vi "ILABs_RemoteCommandHandler.vi"(2 "error In":errorcluster, 4 "data":string, 5 "action":string) -> (0 "errorOut":string, 1 "response":string)   [LabVIEW 2009]
panel:
  out "Control":bool
  out "Connection Status":string
  in  "Case Constant\n(See Context Help)":bool=TRUE
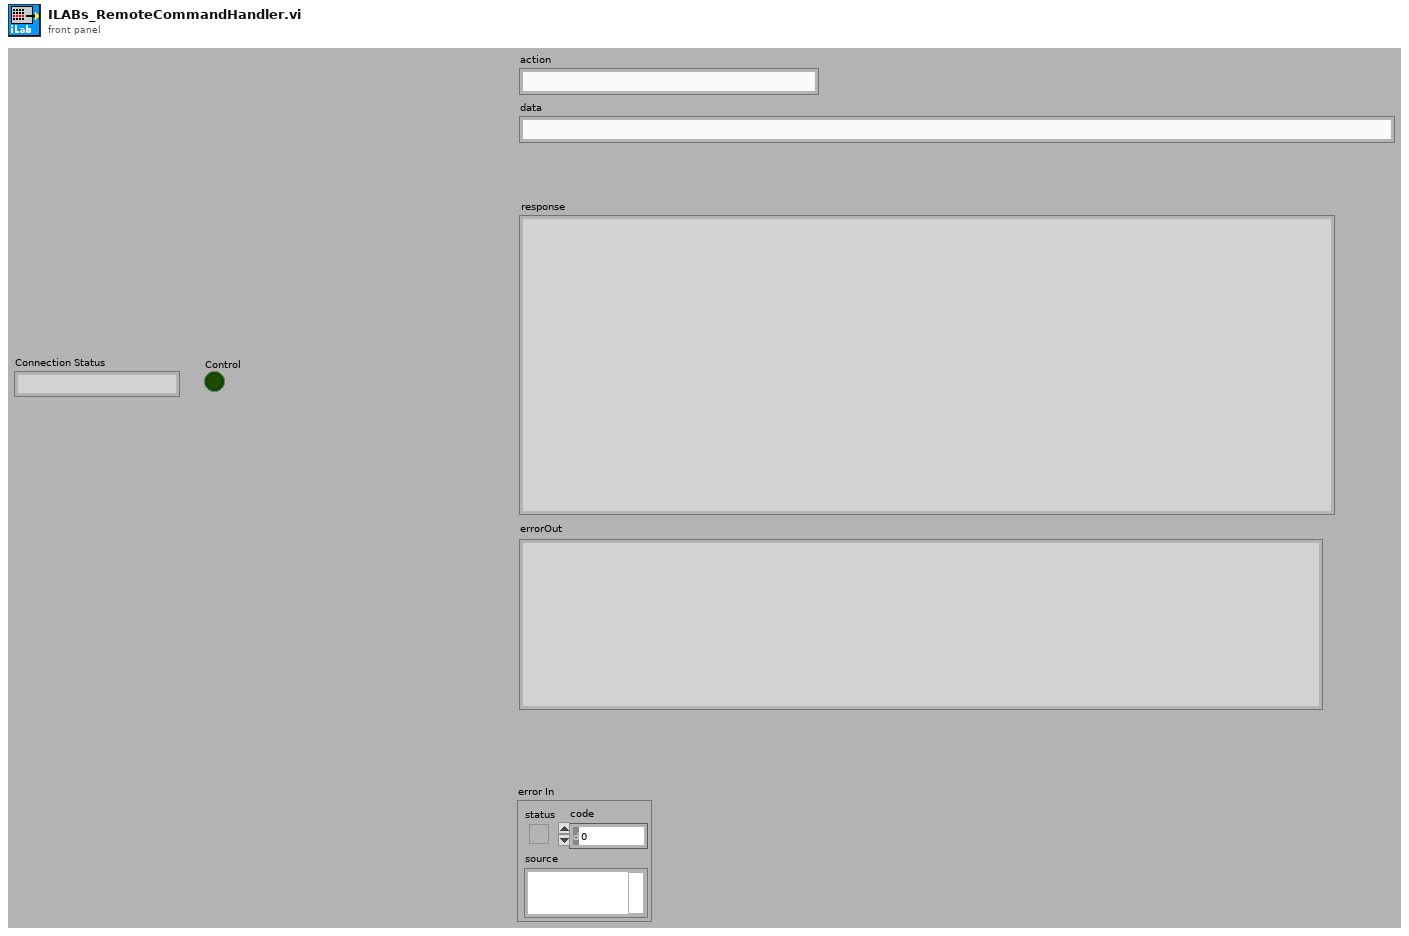
[diagram p1: front panel]
types:
  T1 = typedef "LVRemotePanelConnectionsTypeDef.ctl" = cluster{"VI Name":string, "Remote":string, "UserName":string, "Port":i32, "Status":enum32{"Viewing", "Waiting For Control", "Controlling"}, "Create Time":timestamp, "Status Time":timestamp, "Control End Time":timestamp}[]
  T2 = cluster{"VI Name":string, "Remote":string, "UserName":string, "Port":i32, "Status":enum32{"Viewing", "Waiting For Control", "Controlling"}, "Create Time":timestamp, "Status Time":timestamp, "Control End Time":timestamp}
  T3 = enum32{"Viewing", "Waiting For Control", "Controlling"}
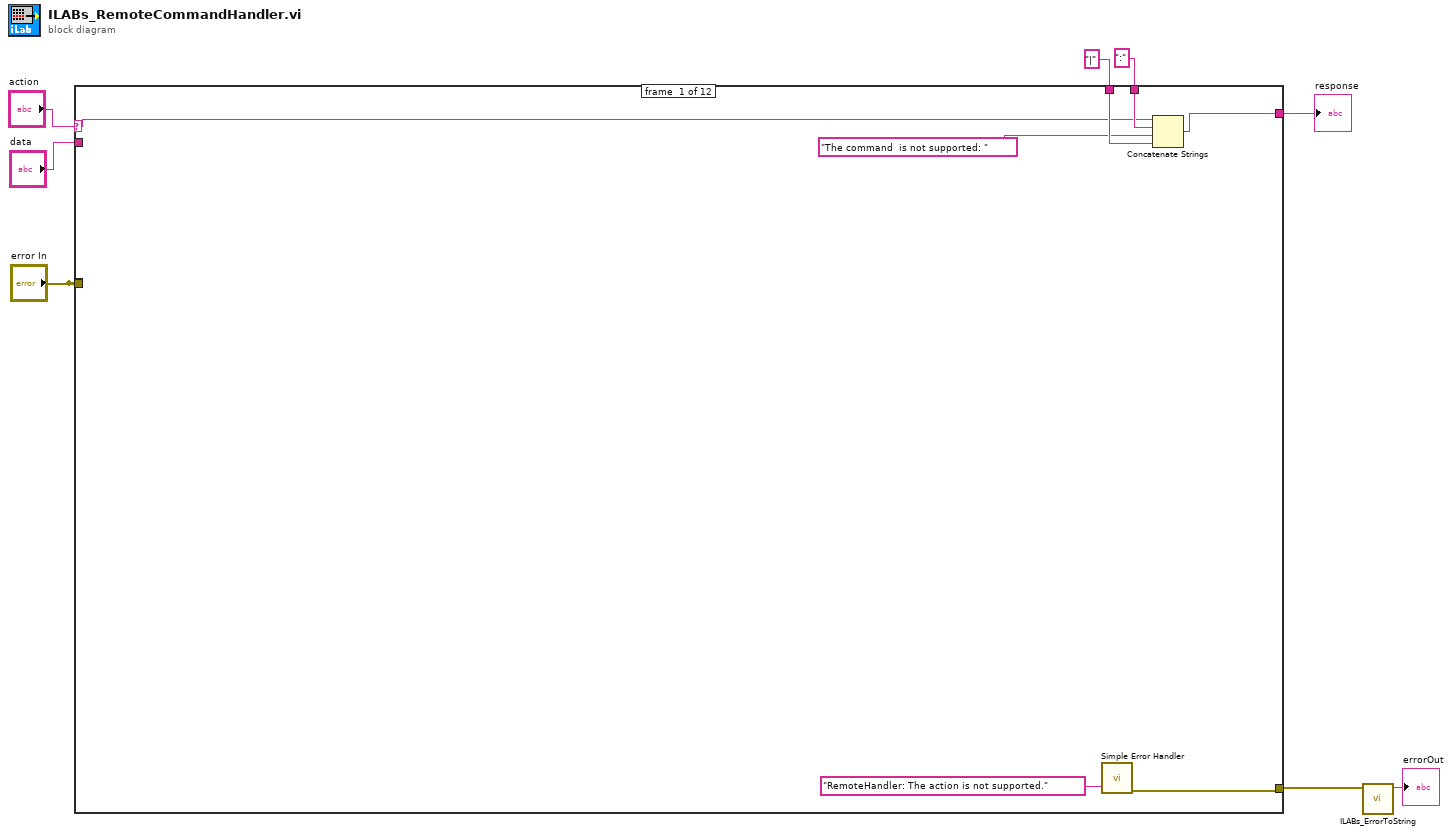
[diagram p0: block diagram]
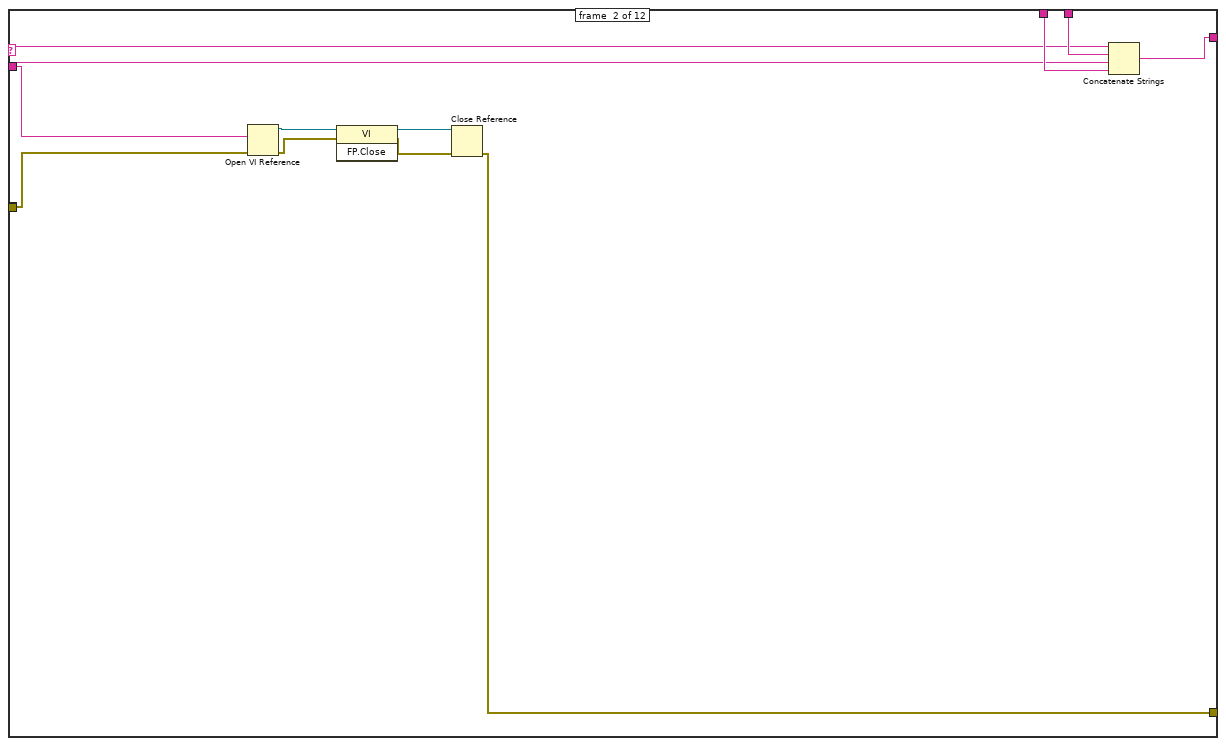
[diagram p2: hidden frame]
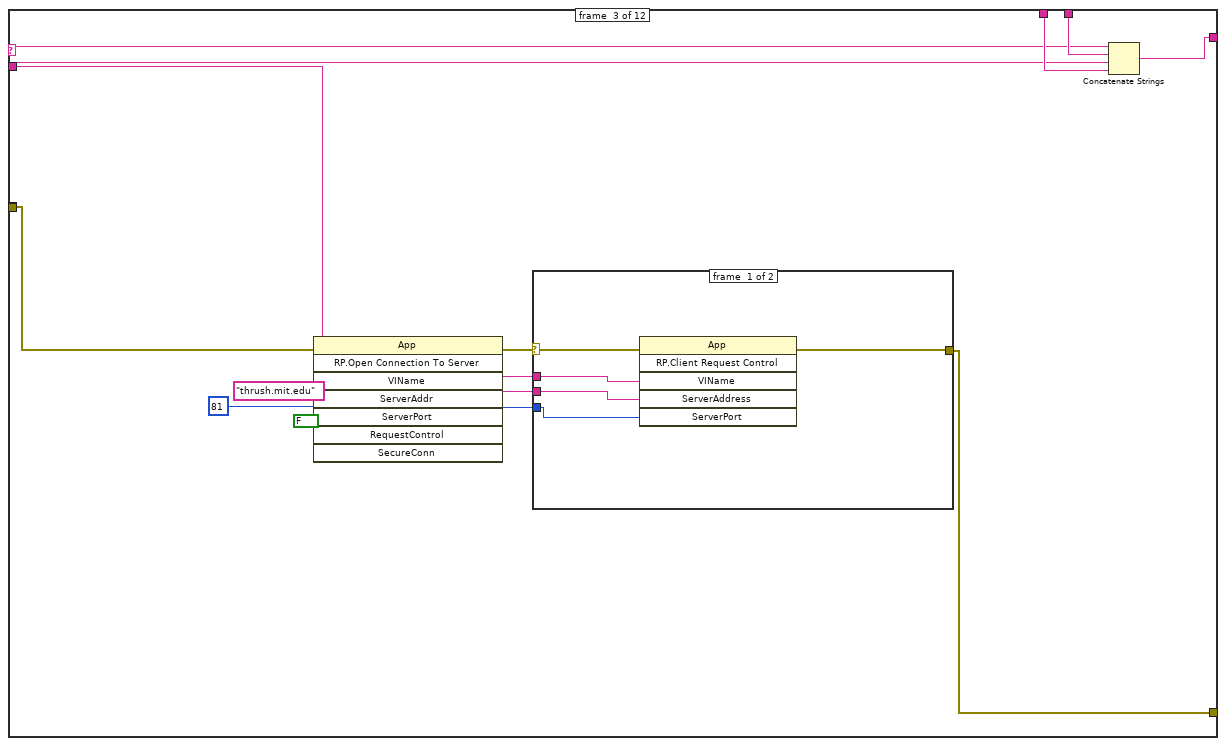
[diagram p3: hidden frame]
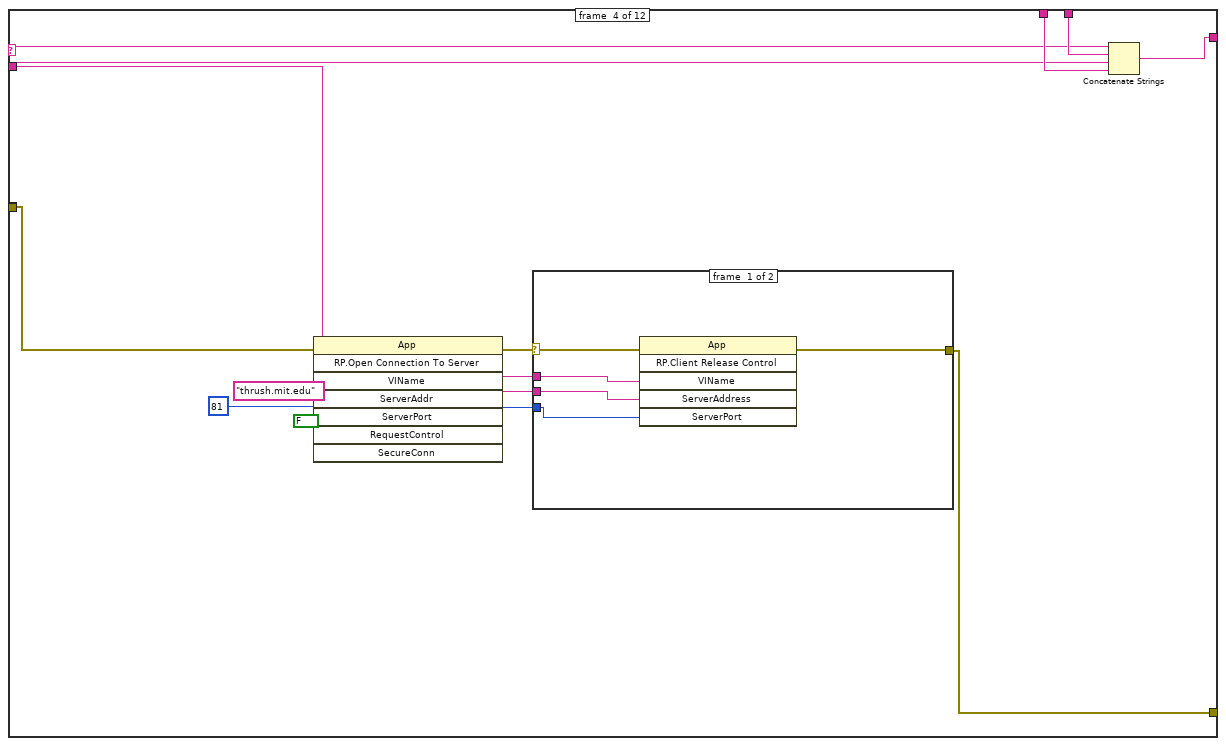
[diagram p5: hidden frame]
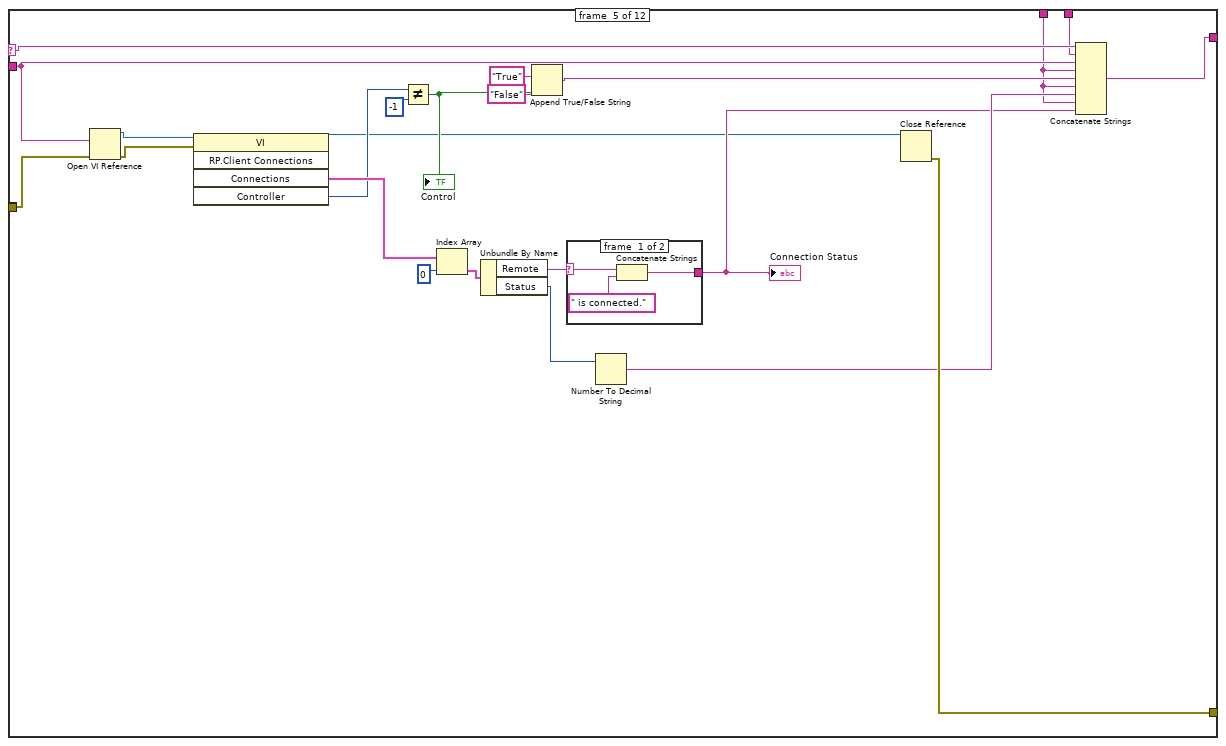
[diagram p7: hidden frame]
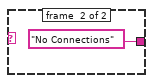
[diagram p8: hidden frame]
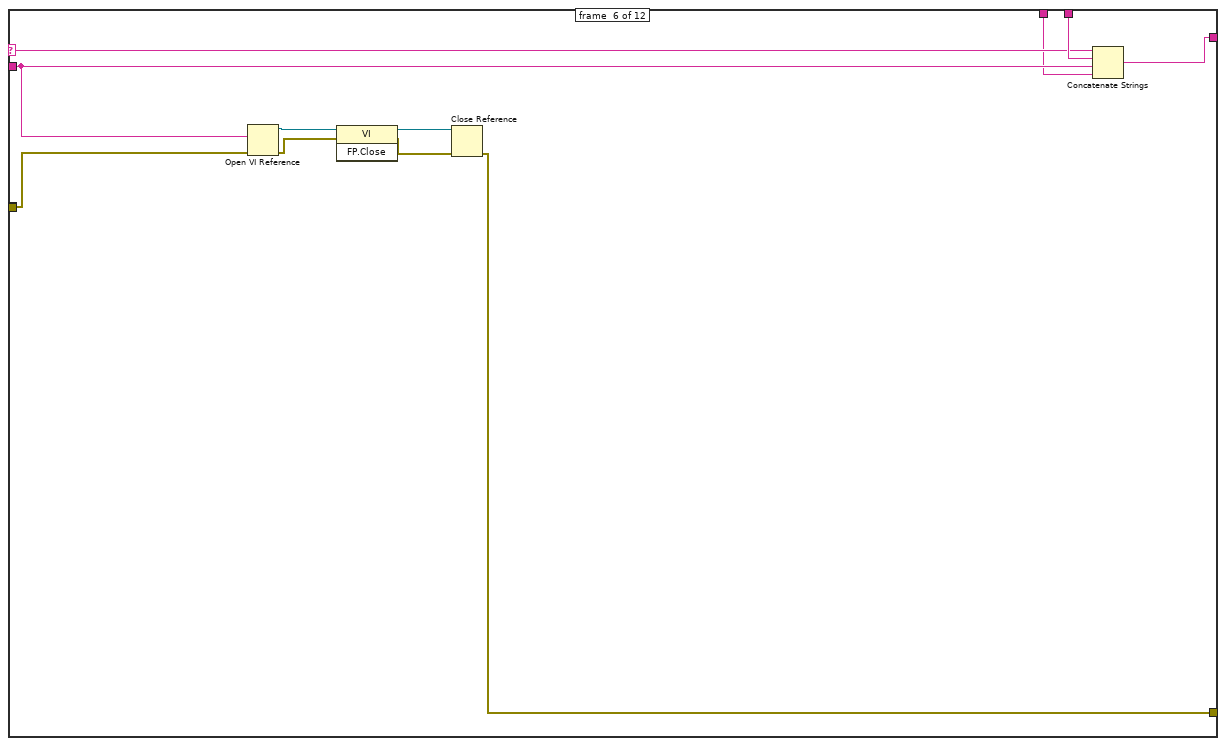
[diagram p9: hidden frame]
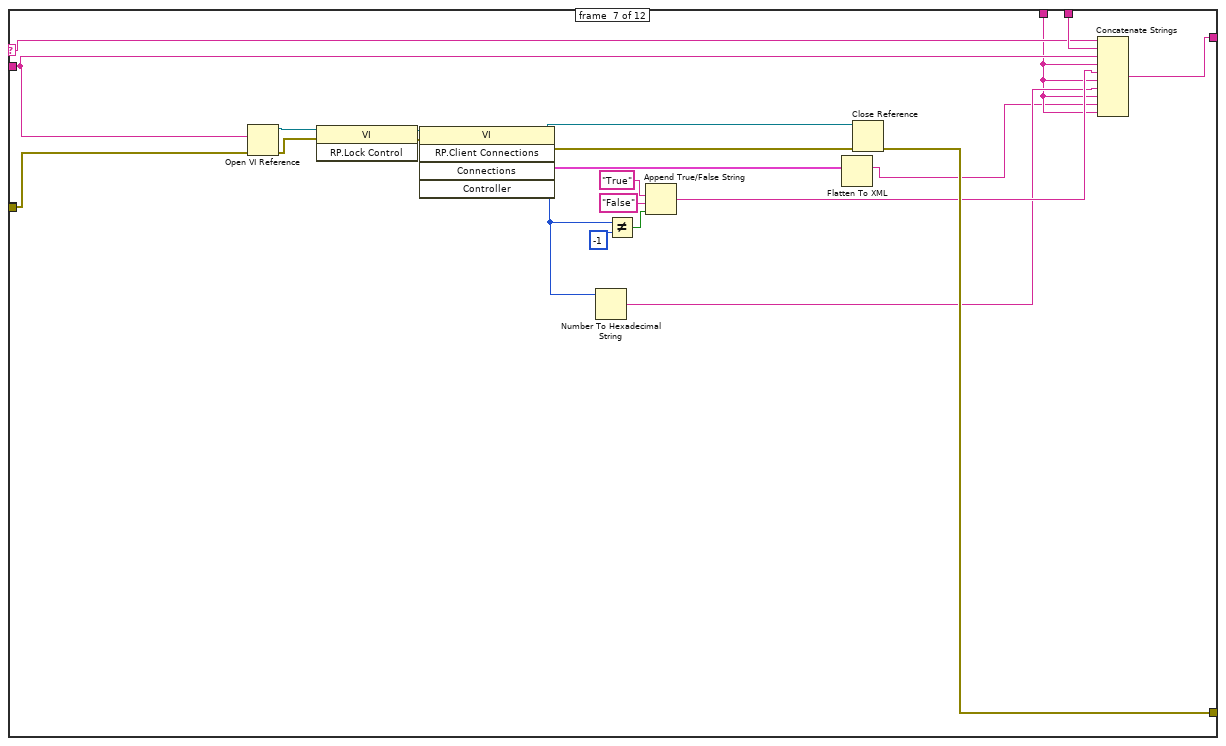
[diagram p10: hidden frame]
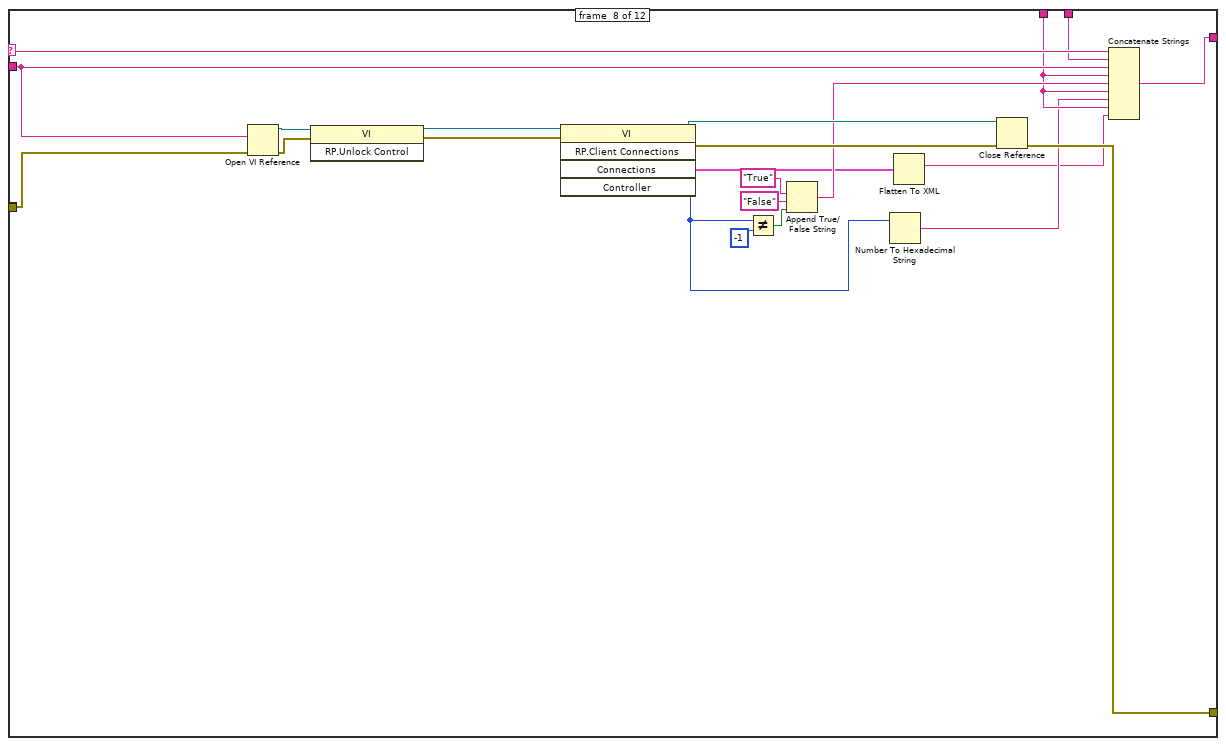
[diagram p11: hidden frame]
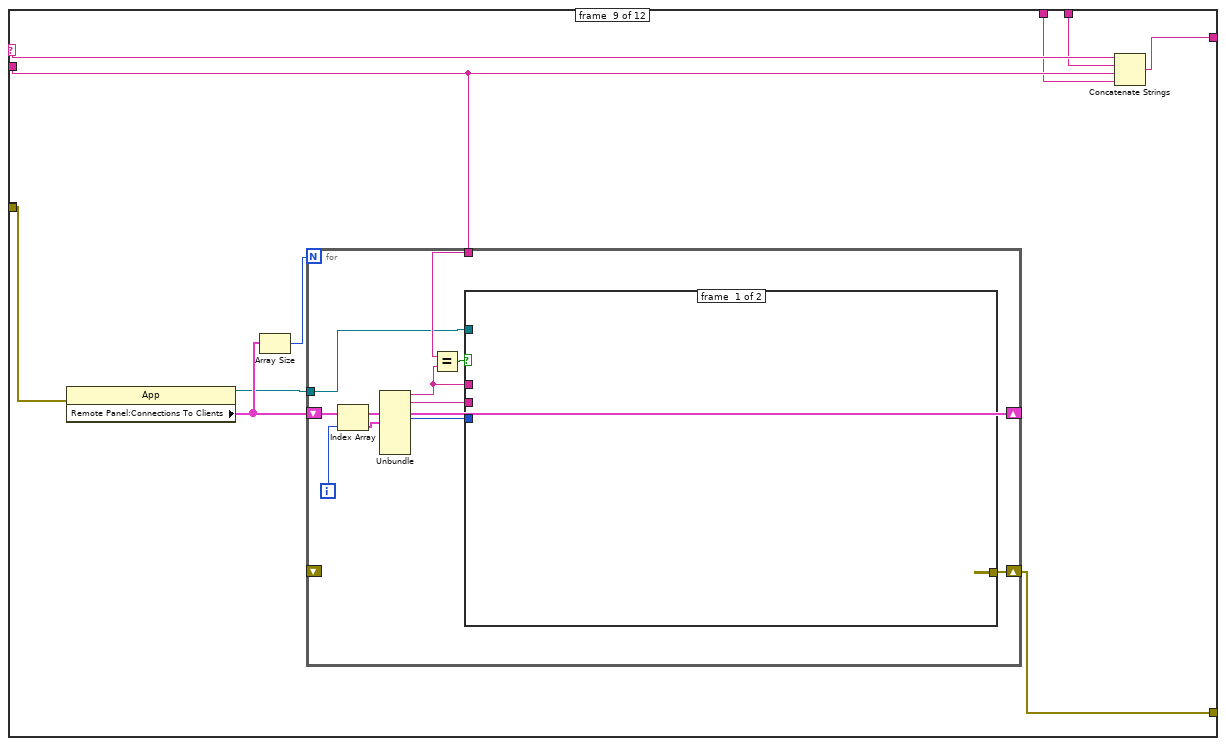
[diagram p12: hidden frame]
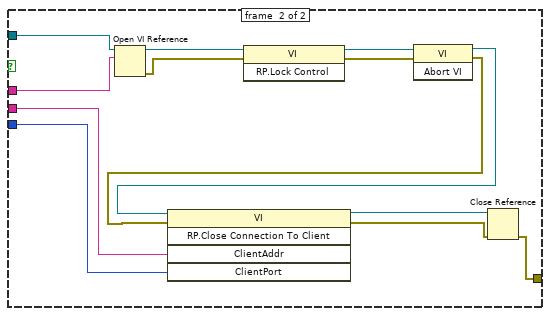
[diagram p13: hidden frame]
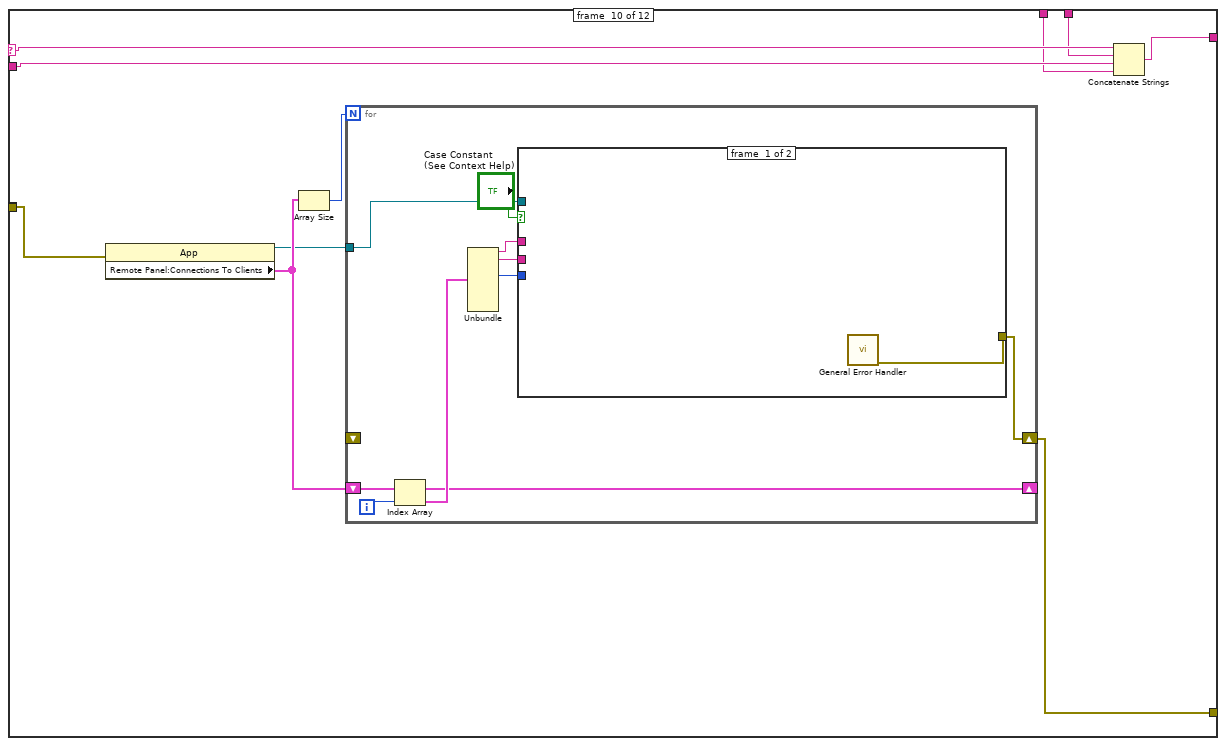
[diagram p14: hidden frame]
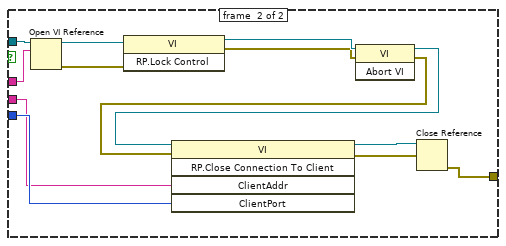
[diagram p15: hidden frame]
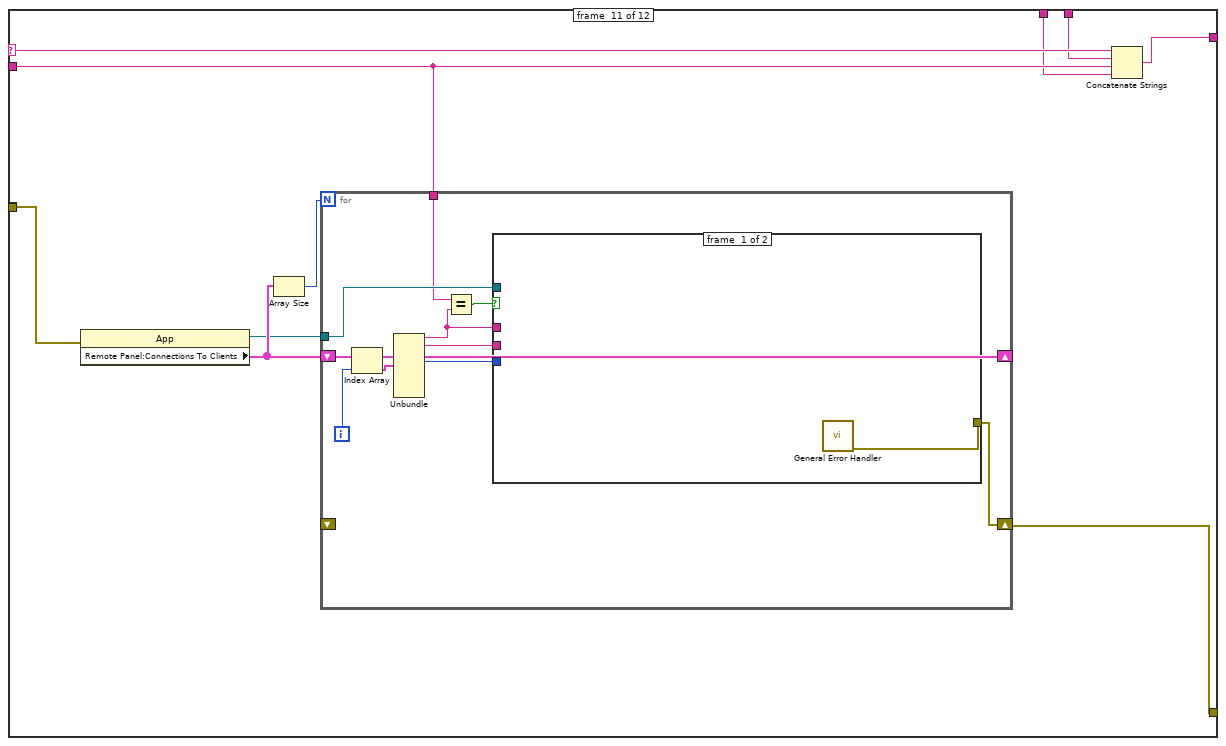
[diagram p16: hidden frame]
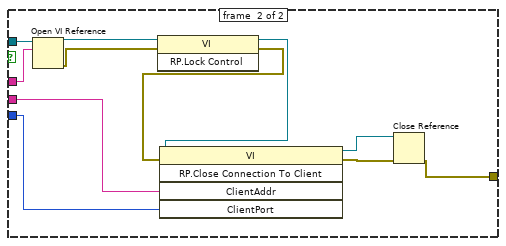
[diagram p17: hidden frame]
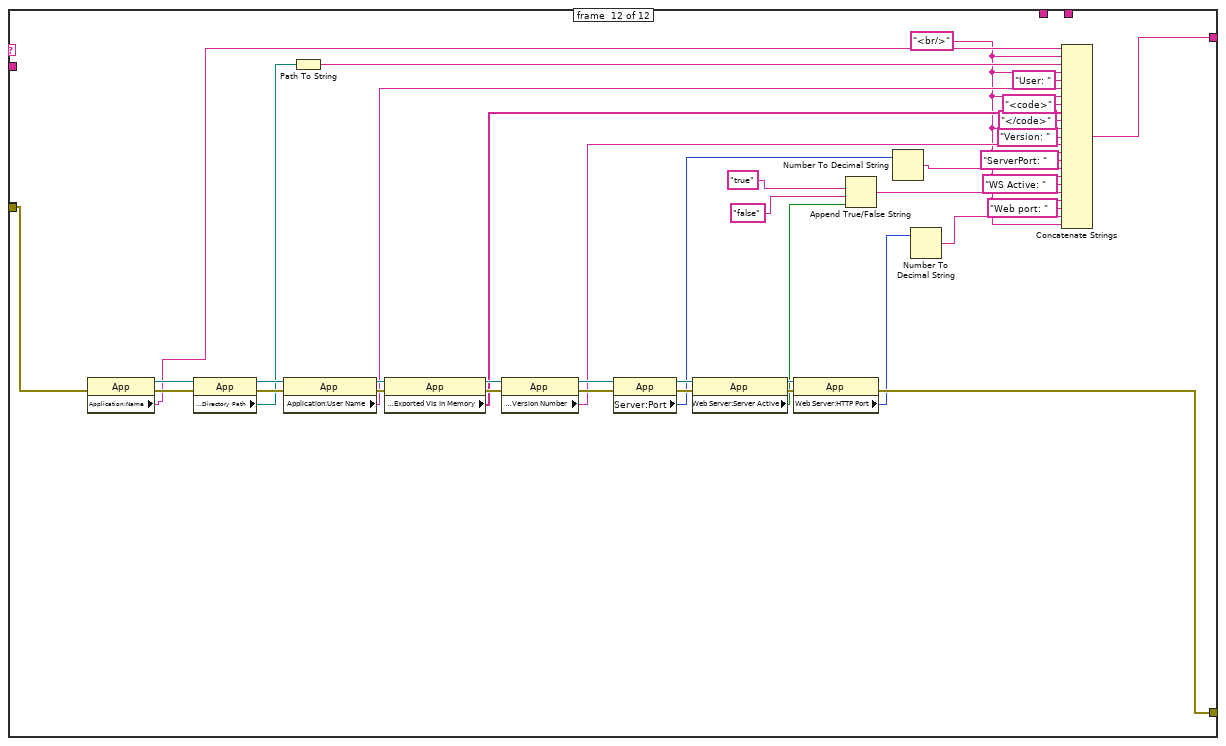
[diagram p18: hidden frame]
diagram:
  n1 = case shown="\"appStatus\"" "action" {
    selector: "action" -> [w9 w17 w34 w51 w67 w90 w107 w129 w146 w179 w212 _]
    tunnel: "data" -> [_ w16 w29 w46 w66 w89 w106 w128 w145 w178 w211 _]
    tunnel: [w15 w20 w37 w54 w81 w92 w116 w138 w152 w183 w218 w241] -> w7
    tunnel: [w13 w21 w28 w45 w82 w93 w117 w139 w147 w182 w213 w264] -> w5
    tunnel: "error In" -> [_ w22 w27 w44 w83 w94 w118 w140 w148 w181 w214 w279]
    tunnel: "error In" -> [_ _ _ _ _ _ _ _ _ _ _ _]
    tunnel: ":" -> [w12 w18 w35 w52 w62 w91 w108 w127 w144 w177 w210 _]
    tunnel: "|" -> [w11 w19 w36 w53 w61 w88 w102 w125 w143 w176 w209 _]
    frame #0 {
      (unwired) "The" ("message")
      n2 = call <vilib>:"Simple Error Handler.vi"("error source (\" \")"="RemoteHandler: The action is not supported." ("error source (\" \")")) -> ("error out"=w13:errorcluster)  [unwired: 2 in, 6 out]
      n3 = Concatenate Strings(w9, w12, "The command  is not supported: " ("string"), w11) -> (w15:string)
    }
    frame #1 {
      n4 = Open VI Reference(vi path=w16, error in (no error)=w22) -> (vi reference=w26:refnum<vi>, error out=w25:errorcluster)  [unwired: 4 out]
      n5 = invoke class="VI" method="FP.Close"(reference=w26, error in=w25) -> (reference out=w24:refnum<vi>, error out=w23:errorcluster)  [unwired: 1 in, 1 out]
      n6 = Close Reference(reference=w24, error in (no error)=w23) -> (error out=w21:errorcluster)
      n7 = Concatenate Strings(w17, w18, w16, w19) -> (w20:string)
    }
    frame #2 {
      w31 = 81 ("Server Port")
      w32 = "thrush.mit.edu" ("Server Address")
      n8 = invoke class="App" method="RP.Open Connection To Server"(error in=w27, "VIName"=w29, "ServerAddr"=w32, "ServerPort"=w31, "RequestControl"=FALSE ("Request Control")) -> (error out=w30:errorcluster)  [unwired: 3 in, 7 out]
      n9 = case shown="No Error" w30 {
        selector: w30 -> [w42 w43]
        tunnel: w29 -> [w41 _]
        tunnel: w32 -> [w40 _]
        tunnel: w31 -> [w39 _]
        tunnel: [w38 w43] -> w28
        frame #0 {
          n10 = invoke class="App" method="RP.Client Request Control"(error in=w42, "VIName"=w41, "ServerAddress"=w40, "ServerPort"=w39) -> (error out=w38:errorcluster)  [unwired: 2 in, 5 out]
        }
        frame #1 {
        }
      }
      n11 = Concatenate Strings(w34, w35, w29, w36) -> (w37:string)
    }
    frame #3 {
      w48 = 81 ("Server Port")
      w49 = "thrush.mit.edu" ("Server Address")
      n12 = invoke class="App" method="RP.Open Connection To Server"(error in=w44, "VIName"=w46, "ServerAddr"=w49, "ServerPort"=w48, "RequestControl"=FALSE ("Request Control")) -> (error out=w47:errorcluster)  [unwired: 3 in, 7 out]
      n13 = case shown="No Error" w47 {
        selector: w47 -> [w59 w60]
        tunnel: w46 -> [w58 _]
        tunnel: w49 -> [w57 _]
        tunnel: w48 -> [w56 _]
        tunnel: [w55 w60] -> w45
        frame #0 {
          n14 = invoke class="App" method="RP.Client Release Control"(error in=w59, "VIName"=w58, "ServerAddress"=w57, "ServerPort"=w56) -> (error out=w55:errorcluster)  [unwired: 2 in, 5 out]
        }
        frame #1 {
        }
      }
      n15 = Concatenate Strings(w51, w52, w46, w53) -> (w54:string)
    }
    frame #4 {
      n16 = Open VI Reference(vi path=w66, error in (no error)=w83) -> (vi reference=w73:refnum<vi>, error out=w74:errorcluster)  [unwired: 4 out]
      n17 = invoke class="VI" method="RP.Client Connections"(reference=w73, error in=w74) -> (reference out=w63:refnum<vi>, "Connections"=w80:T1, "Controller"=w77:i32)  [unwired: 3 in, 2 out]
      n18 = Not Equal?(x=w77, y=-1) -> (x != y?=w72:bool)
      "Control" <- w72
      n19 = Index Array(array=w80, index=0) -> (element=w75:T2)
      n20 = Unbundle By Name(w75) -> ("Remote"=w78:string, "Status"=w68:T3)
      n21 = Append True/False String(1:w72, 2:"False" ("false string"), 3:"True" ("true string")) -> (0:w69:string)  [unwired: 1 out]
      n22 = case shown="\"\"" w78 {
        selector: w78 -> [w86 _]
        tunnel: [w84 "No Connections"] -> w64
        frame #0 {
          n23 = Concatenate Strings(w86, " is connected." ("string")) -> (w84:string)
        }
        frame #1 {
        }
      }
      "Connection Status" <- w64
      n24 = Number To Decimal String(number=w68) -> (decimal integer string=w65:string)  [unwired: 1 out]
      n25 = Close Reference(reference=w63) -> (error out=w82:errorcluster)  [unwired: 1 in]
      n26 = Concatenate Strings(w67, w62, w66, w61, w69, w61, w65, w61, w64) -> (w81:string)
    }
    frame #5 {
      n27 = Open VI Reference(vi path=w89, error in (no error)=w94) -> (vi reference=w98:refnum<vi>, error out=w97:errorcluster)  [unwired: 4 out]
      n28 = invoke class="VI" method="FP.Close"(reference=w98, error in=w97) -> (reference out=w96:refnum<vi>, error out=w95:errorcluster)  [unwired: 1 in, 1 out]
      n29 = Close Reference(reference=w96, error in (no error)=w95) -> (error out=w93:errorcluster)
      n30 = Concatenate Strings(w90, w91, w89, w88) -> (w92:string)
    }
    frame #6 {
      n31 = Open VI Reference(vi path=w106, error in (no error)=w118) -> (vi reference=w120:refnum<vi>, error out=w119:errorcluster)  [unwired: 4 out]
      n32 = invoke class="VI" method="RP.Lock Control"(reference=w120, error in=w119) -> (reference out=w114:refnum<vi>, error out=w113:errorcluster)  [unwired: 1 in, 1 out]
      n33 = invoke class="VI" method="RP.Client Connections"(reference=w114, error in=w113) -> (reference out=w101:refnum<vi>, error out=w115:errorcluster, "Connections"=w99:T1, "Controller"=w104:i32)  [unwired: 3 in, 1 out]
      n34 = Number To Hexadecimal String(2:w104) -> (0:w103:string)  [unwired: 1 out]
      n35 = Not Equal?(x=w104, y=-1) -> (x != y?=w111:bool)
      n36 = Append True/False String(1:w111, 2:"False" ("false string"), 3:"True" ("true string")) -> (0:w105:string)  [unwired: 1 out]
      n37 = Flatten To XML(anything=w99) -> (xml string=w100:string)
      n38 = Close Reference(reference=w101, error in (no error)=w115) -> (error out=w117:errorcluster)
      n39 = Concatenate Strings(w107, w108, w106, w102, w105, w102, w103, w102, w100, w102) -> (w116:string)
    }
    frame #7 {
      n40 = Open VI Reference(vi path=w128, error in (no error)=w140) -> (vi reference=w142:refnum<vi>, error out=w141:errorcluster)  [unwired: 4 out]
      n41 = invoke class="VI" method="RP.Unlock Control"(reference=w142, error in=w141) -> (reference out=w131:refnum<vi>, error out=w130:errorcluster)  [unwired: 1 in, 1 out]
      n42 = invoke class="VI" method="RP.Client Connections"(reference=w131, error in=w130) -> (reference out=w132:refnum<vi>, error out=w133:errorcluster, "Connections"=w122:T1, "Controller"=w124:i32)  [unwired: 3 in, 1 out]
      n43 = Not Equal?(x=w124, y=-1) -> (x != y?=w136:bool)
      n44 = Append True/False String(1:w136, 2:"False" ("false string"), 3:"True" ("true string")) -> (0:w126:string)  [unwired: 1 out]
      n45 = Number To Hexadecimal String(2:w124) -> (0:w123:string)  [unwired: 1 out]
      n46 = Flatten To XML(anything=w122) -> (xml string=w121:string)
      n47 = Close Reference(reference=w132, error in (no error)=w133) -> (error out=w139:errorcluster)
      n48 = Concatenate Strings(w129, w127, w128, w125, w126, w125, w123, w125, w121) -> (w138:string)
    }
    frame #8 {
      n49 = property class="App"(error in=w148) -> (reference out=w149:refnum<vi>, "Remote Panel:Connections To Clients"=w150:T1)  [unwired: 1 in, 1 out]
      n50 = Array Size(array=w150) -> (size(s)=w151:i32)
      n51 = for {
        N: w151 -> [_]
        shift-right: [w154] -> _
        shift-left: w150 -> [w154]
        tunnel: w145 -> [w160]
        shift-right: [w156] -> w147
        shift-left: _ -> [_]
        tunnel: w149 -> [w153]
        i -> [w162]
        n52 = Index Array(array=w154, index=w162) -> (element=w161:T2)
        n53 = Unbundle(w161) -> ("VI Name"=w155:string, "Remote"=w157:string, "Port"=w158:i32)  [unwired: 5 out]
        n54 = Equal?(x=w160, y=w155) -> (x = y?=w159:bool)
        n55 = case shown="True" w159 {
          tunnel: w158 -> [_ w175]
          tunnel: w157 -> [_ w174]
          tunnel: [_ w173] -> w156
          tunnel: w155 -> [_ w172]
          tunnel: w153 -> [_ w163]
          frame #0 {
          }
          frame #1 {
            n56 = Open VI Reference(application reference (local)=w163, vi path=w172) -> (vi reference=w171:refnum<vi>, error out=w170:errorcluster)  [unwired: 1 in, 3 out]
            n57 = invoke class="VI" method="RP.Lock Control"(reference=w171, error in=w170) -> (reference out=w169:refnum<vi>, error out=w168:errorcluster)  [unwired: 1 in, 1 out]
            n58 = invoke class="VI" method="Abort VI"(reference=w169, error in=w168) -> (reference out=w165:refnum<vi>, error out=w167:errorcluster)  [unwired: 1 in, 1 out]
            n59 = invoke class="VI" method="RP.Close Connection To Client"(reference=w165, error in=w167, "ClientAddr"=w174, "ClientPort"=w175) -> (reference out=w164:refnum<vi>, error out=w166:errorcluster)  [unwired: 1 in, 3 out]
            n60 = Close Reference(reference=w164, error in (no error)=w166) -> (error out=w173:errorcluster)
          }
        }
      }
      n61 = Concatenate Strings(w146, w144, w145, w143) -> (w152:string)
    }
    frame #9 {
      n62 = property class="App"(error in=w181) -> (reference out=w180:refnum<vi>, "Remote Panel:Connections To Clients"=w184:T1)  [unwired: 1 in, 1 out]
      n63 = Array Size(array=w184) -> (size(s)=w185:i32)
      n64 = for {
        N: w185 -> [_]
        shift-right: [w188] -> _
        shift-left: w184 -> [w188]
        shift-right: [w190] -> w182
        shift-left: _ -> [_]
        tunnel: w180 -> [w186]
        i -> [w194]
        n65 = Index Array(array=w188, index=w194) -> (element=w193:T2)
        n66 = Unbundle(w193) -> ("VI Name"=w189:string, "Remote"=w191:string, "Port"=w192:i32)  [unwired: 5 out]
        n67 = case shown="True" "Case Constant\n(See Context Help)" {
          tunnel: w192 -> [_ w208]
          tunnel: w191 -> [_ w207]
          tunnel: [w195 w206] -> w190
          tunnel: w189 -> [_ w205]
          tunnel: w186 -> [_ w196]
          frame #0 {
            n68 = call <vilib>:"General Error Handler.vi"() -> ("error out"=w195:errorcluster)  [unwired: 2 in, 13 out]
          }
          frame #1 {
            n69 = Open VI Reference(application reference (local)=w196, vi path=w205) -> (vi reference=w200:refnum<vi>, error out=w199:errorcluster)  [unwired: 1 in, 3 out]
            n70 = invoke class="VI" method="RP.Lock Control"(reference=w200, error in=w199) -> (reference out=w198:refnum<vi>, error out=w197:errorcluster)  [unwired: 1 in, 1 out]
            n71 = invoke class="VI" method="Abort VI"(reference=w198, error in=w197) -> (reference out=w201:refnum<vi>, error out=w202:errorcluster)  [unwired: 1 in, 1 out]
            n72 = invoke class="VI" method="RP.Close Connection To Client"(reference=w201, error in=w202, "ClientAddr"=w207, "ClientPort"=w208) -> (reference out=w204:refnum<vi>, error out=w203:errorcluster)  [unwired: 1 in, 3 out]
            n73 = Close Reference(reference=w204, error in (no error)=w203) -> (error out=w206:errorcluster)
          }
        }
      }
      n74 = Concatenate Strings(w179, w177, w178, w176) -> (w183:string)
    }
    frame #10 {
      n75 = property class="App"(error in=w214) -> (reference out=w215:refnum<vi>, "Remote Panel:Connections To Clients"=w216:T1)  [unwired: 1 in, 1 out]
      n76 = Array Size(array=w216) -> (size(s)=w217:i32)
      n77 = for {
        N: w217 -> [_]
        shift-right: [w221] -> _
        shift-left: w216 -> [w221]
        tunnel: w211 -> [w219]
        shift-right: [w223] -> w213
        shift-left: _ -> [_]
        tunnel: w215 -> [w220]
        i -> [w228]
        n78 = Index Array(array=w221, index=w228) -> (element=w227:T2)
        n79 = Unbundle(w227) -> ("VI Name"=w222:string, "Remote"=w224:string, "Port"=w225:i32)  [unwired: 5 out]
        n80 = Equal?(x=w219, y=w222) -> (x = y?=w226:bool)
        n81 = case shown="True" w226 {
          tunnel: w225 -> [_ w240]
          tunnel: w224 -> [_ w239]
          tunnel: [w229 w230] -> w223
          tunnel: w222 -> [_ w238]
          tunnel: w220 -> [_ w233]
          frame #0 {
            n82 = call <vilib>:"General Error Handler.vi"() -> ("error out"=w229:errorcluster)  [unwired: 2 in, 13 out]
          }
          frame #1 {
            n83 = Open VI Reference(application reference (local)=w233, vi path=w238) -> (vi reference=w237:refnum<vi>, error out=w234:errorcluster)  [unwired: 1 in, 3 out]
            n84 = invoke class="VI" method="RP.Lock Control"(reference=w237, error in=w234) -> (reference out=w236:refnum<vi>, error out=w235:errorcluster)  [unwired: 1 in, 1 out]
            n85 = invoke class="VI" method="RP.Close Connection To Client"(reference=w236, error in=w235, "ClientAddr"=w239, "ClientPort"=w240) -> (reference out=w231:refnum<vi>, error out=w232:errorcluster)  [unwired: 1 in, 3 out]
            n86 = Close Reference(reference=w231, error in (no error)=w232) -> (error out=w230:errorcluster)
          }
        }
      }
      n87 = Concatenate Strings(w212, w210, w211, w209) -> (w218:string)
    }
    frame #11 {
      w242 = "<br/>" ("string")
      n88 = property class="App"(error in=w279) -> (reference out=w278:refnum<vi>, error out=w273:errorcluster, "Application:Name"=w263:string)  [unwired: 1 in]
      n89 = property class="App"(reference=w278, error in=w273) -> (reference out=w277:refnum<vi>, error out=w272:errorcluster, "Application:Directory Path"=w261:path)
      n90 = property class="App"(reference=w277, error in=w272) -> (reference out=w276:refnum<vi>, error out=w271:errorcluster, "Application:User Name"=w259:string)
      n91 = Path To String(path=w261) -> (string=w262:string)
      n92 = property class="App"(reference=w276, error in=w271) -> (reference out=w275:refnum<vi>, error out=w270:errorcluster, "Application:Exported VIs In Memory"=w257:string[])
      n93 = property class="App"(reference=w275, error in=w270) -> (reference out=w274:refnum<vi>, error out=w269:errorcluster, "Application:Version Number"=w254:string)
      n94 = property class="App"(reference=w274, error in=w269) -> (reference out=w265:refnum<vi>, error out=w266:errorcluster, "Server:Port"=w251:u32)
      n95 = property class="App"(reference=w265, error in=w266) -> (reference out=w268:refnum<vi>, error out=w267:errorcluster, "Web Server:Server Active"=w249:bool)
      n96 = property class="App"(reference=w268, error in=w267) -> (error out=w264:errorcluster, "Web Server:HTTP Port"=w244:u16)  [unwired: 1 out]
      n97 = Append True/False String(1:w249, 2:"false" ("false string"), 3:"true" ("true string")) -> (0:w248:string)  [unwired: 1 out]
      n98 = Number To Decimal String(number=w251) -> (decimal integer string=w252:string)  [unwired: 1 out]
      n99 = Number To Decimal String(number=w244) -> (decimal integer string=w243:string)  [unwired: 1 out]
      n100 = Concatenate Strings(w263, w242, w262, w242, "User: " ("string"), w259, w242, "<code>" ("string"), w257, "</code>" ("string"), w242, "Version: " ("string"), w254, w242, "ServerPort: " ("string"), w252, w242, "WS Active: " ("string"), w248, w242, "Web port: " ("string"), w243, w242) -> (w241:string)
    }
  }
  "response" <- w7
  n101 = call "ILABs_ErrorToString.vi"("errorIn"=w5) -> ("errorOut"=→"errorOut":string)  [unwired: 10 out]
